vi "功能试验判定.vi"(7 "Result":refnum<vi>, 10 "判定参数":T1, 11 "XY曲线":cluster{"X":dbl[], "Y":dbl[]}[](array[cluster])) -> (2 "判定项长度":i32, 3 "OK？":bool)   [LabVIEW 2020]
uses:
  <userlib>/_MGI/1D Array/MGI Average/MGI Average (DBL[]).vi
panel:
  out "逆向平均值":dbl
  out "正向平均值":dbl
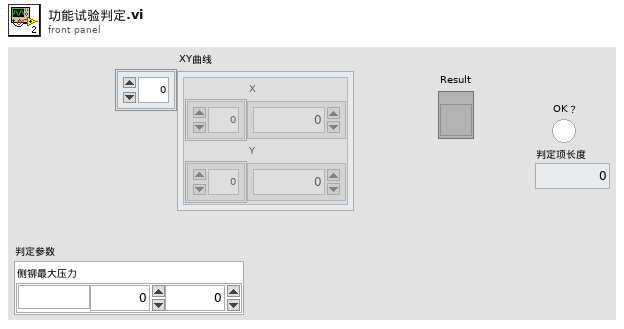
[diagram p1: front panel]
types:
  T1 = cluster{"侧铆最大压力":cluster{"单位":string, "下限":dbl, "上限":dbl}}
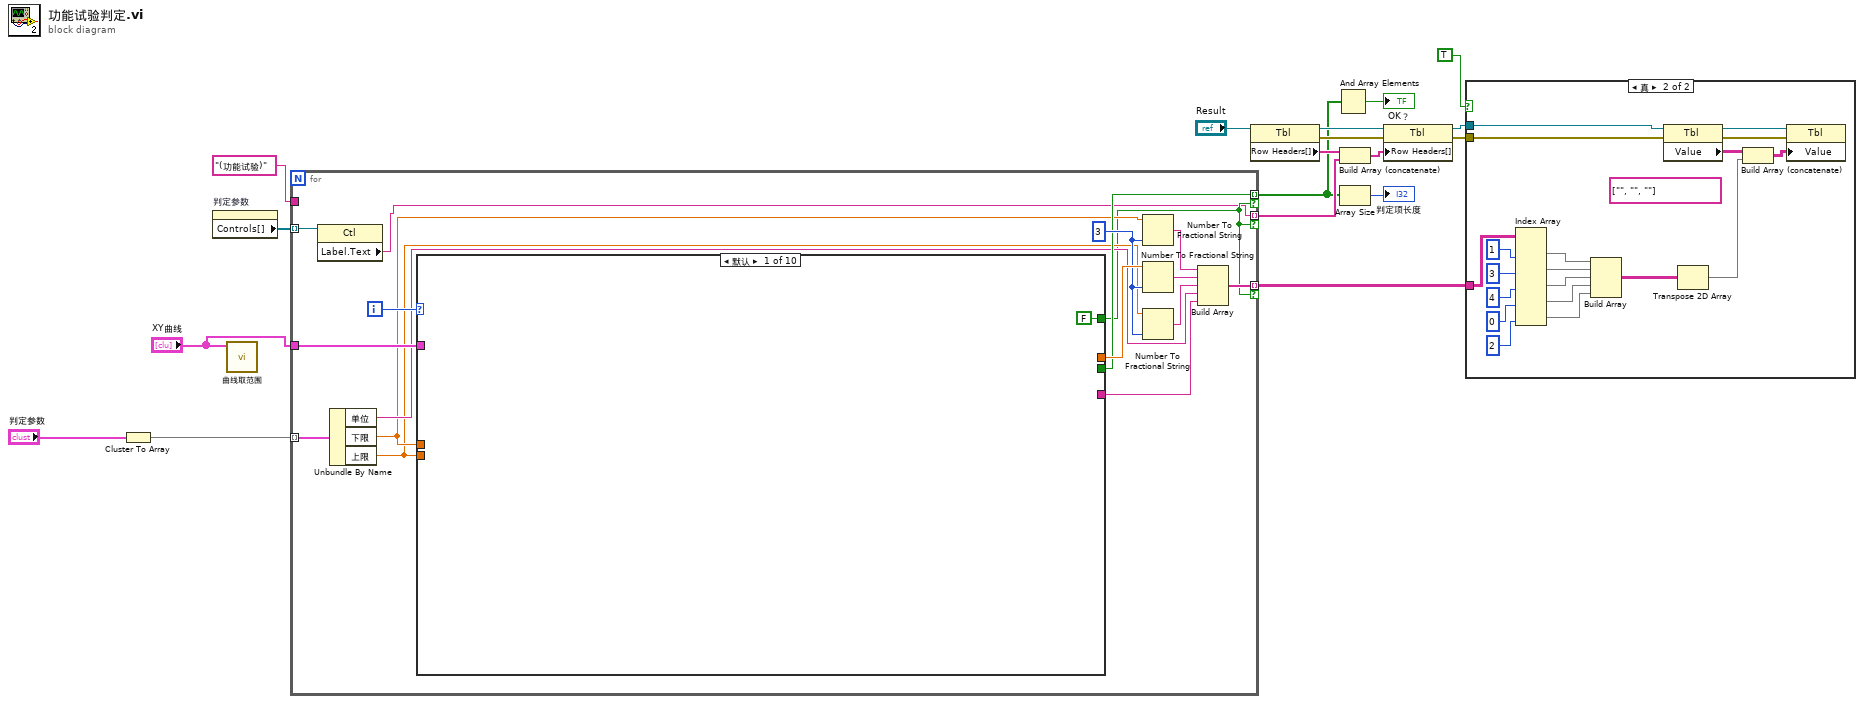
[diagram p0: block diagram]
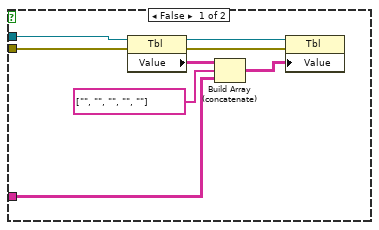
[diagram p2: hidden frame]
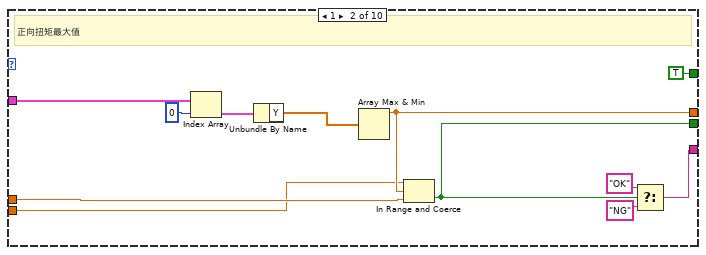
[diagram p3: hidden frame]
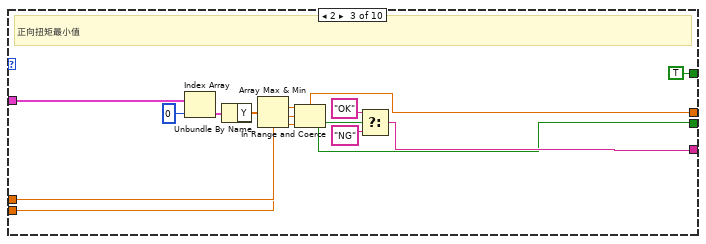
[diagram p4: hidden frame]
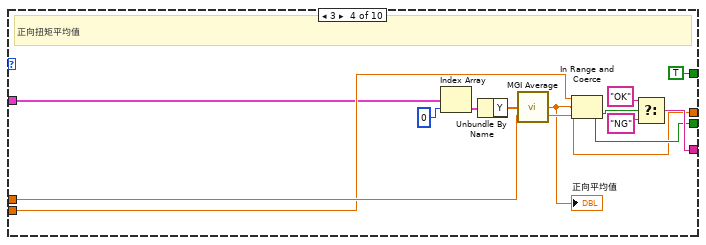
[diagram p5: hidden frame]
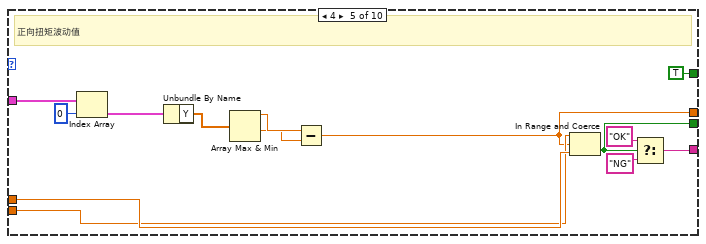
[diagram p6: hidden frame]
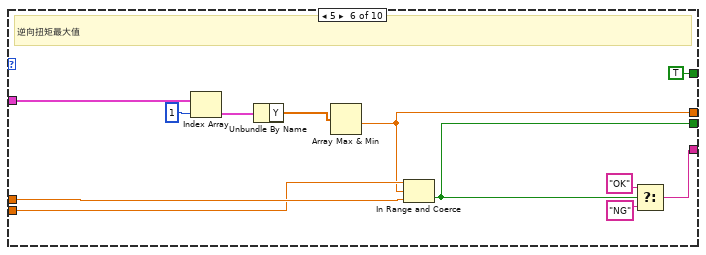
[diagram p7: hidden frame]
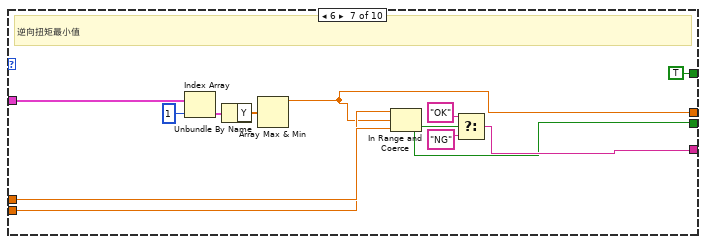
[diagram p8: hidden frame]
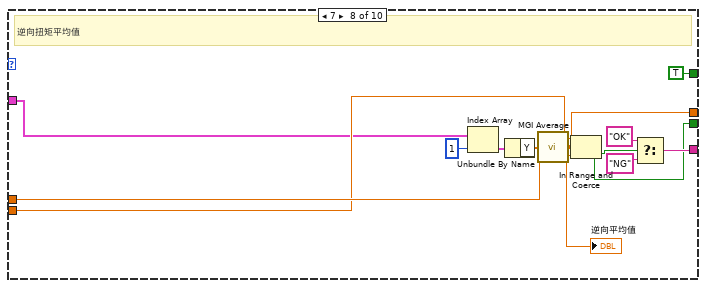
[diagram p9: hidden frame]
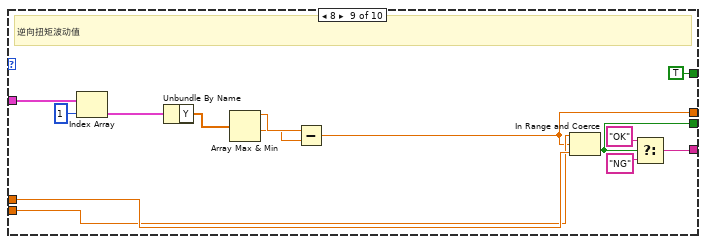
[diagram p10: hidden frame]
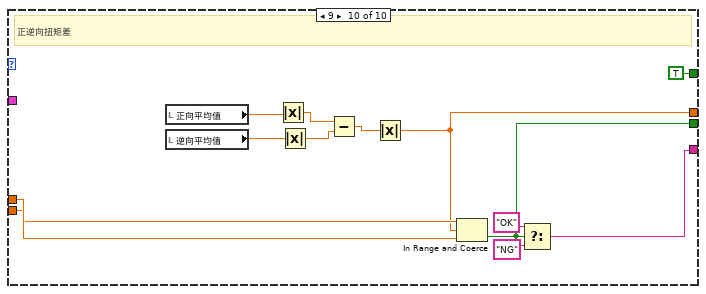
[diagram p11: hidden frame]
diagram:
  n1 = Cluster To Array(cluster="判定参数") -> (array=w18:cluster{"单位":string, "下限":dbl, "上限":dbl}[])
  n2 = property on="判定参数" class="Clust (严格)"() -> ("Controls[]"=w7:refnum<vi>[])  [unwired: 2 in, 2 out]
  n3 = call "曲线取范围.vi"("曲线In"="XY曲线") -> ()  [unwired: 10 in, 1 out]
  n4 = for {
    tunnel: w18 -> [w35] mode=indexing
    tunnel: w7 -> [w33] mode=indexing
    tunnel: "XY曲线" -> [w31]
    tunnel: [w25] -> w5 mode=indexing if=w20
    tunnel: [w21] -> w8 mode=indexing if=w20
    tunnel: [w19] -> w11 mode=indexing if=w20
    tunnel: "(功能试验)" ("Label.Text") -> [_]
    i -> [w34]
    w30 = i16 3 ("精度(6)")
    n5 = property class="Ctl"(reference=w33) -> ("Label.Text"=w19:string)  [unwired: 1 in, 2 out]
    n6 = Unbundle By Name(w35) -> ("单位"=w24:string, "下限"=w23:dbl, "上限"=w22:dbl)
    n7 = case shown="默认" w34 {
      tunnel: [_ w45 w51 w61 w73 w87 w99 w111 w123 w137] -> w32
      tunnel: w31 -> [_ w48 w60 w65 w79 w98 w110 w115 w129 _]
      tunnel: [_ w42 w56 w70 w84 w93 w106 w120 w134 w139] -> w26
      tunnel: [_ w41 w55 w69 w83 w92 w105 w119 w133 w138] -> w25
      tunnel: w23 -> [_ w40 w54 w68 w82 w91 w104 w118 w132 w146]
      tunnel: w22 -> [_ w39 w53 w67 w81 w90 w103 w117 w131 w145]
      tunnel: [FALSE TRUE TRUE TRUE TRUE TRUE TRUE TRUE TRUE TRUE] -> w20
      frame Default {
      }
      frame 1 {
        # "正向扭矩最大值"
        n8 = Index Array(array=w48, index=0 ("索引")) -> (element=w46:cluster{"X":dbl[], "Y":dbl[]})
        n9 = Unbundle By Name(w46) -> ("Y"=w37:dbl[])
        n10 = Array Max & Min(array=w37) -> (max value=w45:dbl)  [unwired: 3 out]
        n11 = In Range and Coerce(upper limit=w39, x=w45, lower limit=w40) -> (In Range?=w41:bool)  [unwired: 1 out]
        n12 = Select(t="OK", s=w41, f="NG") -> (s? t:f=w42:string)
      }
      frame 2 {
        # "正向扭矩最小值"
        n13 = Index Array(array=w60, index=0 ("索引")) -> (element=w59:cluster{"X":dbl[], "Y":dbl[]})
        n14 = Unbundle By Name(w59) -> ("Y"=w50:dbl[])
        n15 = Array Max & Min(array=w50) -> (min value=w51:dbl)  [unwired: 3 out]
        n16 = In Range and Coerce(upper limit=w53, x=w51, lower limit=w54) -> (In Range?=w55:bool)  [unwired: 1 out]
        n17 = Select(t="OK", s=w55, f="NG") -> (s? t:f=w56:string)
      }
      frame 3 {
        # "正向扭矩平均值"
        n18 = Index Array(array=w65, index=0 ("索引")) -> (element=w64:cluster{"X":dbl[], "Y":dbl[]})
        n19 = Unbundle By Name(w64) -> ("Y"=w63:dbl[])
        n20 = call-poly <userlib>:"MGI Average.vi"("Double[]"=w63) -> ("Average"=w61:dbl)  [unwired: 1 in]
        "正向平均值" <- w61
        n21 = In Range and Coerce(upper limit=w67, x=w61, lower limit=w68) -> (In Range?=w69:bool)  [unwired: 1 out]
        n22 = Select(t="OK", s=w69, f="NG") -> (s? t:f=w70:string)
      }
      frame 4 {
        # "正向扭矩波动值"
        n23 = Index Array(array=w79, index=0 ("索引")) -> (element=w78:cluster{"X":dbl[], "Y":dbl[]})
        n24 = Unbundle By Name(w78) -> ("Y"=w76:dbl[])
        n25 = Array Max & Min(array=w76) -> (max value=w75:dbl, min value=w74:dbl)  [unwired: 2 out]
        n26 = Subtract(x=w75, y=w74) -> (x-y=w73:dbl)
        n27 = In Range and Coerce(upper limit=w81, x=w73, lower limit=w82) -> (In Range?=w83:bool)  [unwired: 1 out]
        n28 = Select(t="OK", s=w83, f="NG") -> (s? t:f=w84:string)
      }
      frame 5 {
        # "逆向扭矩最大值"
        n29 = Index Array(array=w98, index=1 ("索引")) -> (element=w96:cluster{"X":dbl[], "Y":dbl[]})
        n30 = Unbundle By Name(w96) -> ("Y"=w88:dbl[])
        n31 = Array Max & Min(array=w88) -> (min value=w87:dbl)  [unwired: 3 out]
        n32 = In Range and Coerce(upper limit=w90, x=w87, lower limit=w91) -> (In Range?=w92:bool)  [unwired: 1 out]
        n33 = Select(t="OK", s=w92, f="NG") -> (s? t:f=w93:string)
      }
      frame 6 {
        # "逆向扭矩最小值"
        n34 = Index Array(array=w110, index=1 ("索引")) -> (element=w109:cluster{"X":dbl[], "Y":dbl[]})
        n35 = Unbundle By Name(w109) -> ("Y"=w101:dbl[])
        n36 = Array Max & Min(array=w101) -> (max value=w99:dbl)  [unwired: 3 out]
        n37 = In Range and Coerce(upper limit=w103, x=w99, lower limit=w104) -> (In Range?=w105:bool)  [unwired: 1 out]
        n38 = Select(t="OK", s=w105, f="NG") -> (s? t:f=w106:string)
      }
      frame 7 {
        # "逆向扭矩平均值"
        n39 = Index Array(array=w115, index=1 ("索引")) -> (element=w114:cluster{"X":dbl[], "Y":dbl[]})
        n40 = Unbundle By Name(w114) -> ("Y"=w113:dbl[])
        n41 = call-poly <userlib>:"MGI Average.vi"("Double[]"=w113) -> ("Average"=w111:dbl)  [unwired: 1 in]
        "逆向平均值" <- w111
        n42 = In Range and Coerce(upper limit=w117, x=w111, lower limit=w118) -> (In Range?=w119:bool)  [unwired: 1 out]
        n43 = Select(t="OK", s=w119, f="NG") -> (s? t:f=w120:string)
      }
      frame 8 {
        # "逆向扭矩波动值"
        n44 = Index Array(array=w129, index=1 ("索引")) -> (element=w128:cluster{"X":dbl[], "Y":dbl[]})
        n45 = Unbundle By Name(w128) -> ("Y"=w126:dbl[])
        n46 = Array Max & Min(array=w126) -> (max value=w125:dbl, min value=w124:dbl)  [unwired: 2 out]
        n47 = Subtract(x=w125, y=w124) -> (x-y=w123:dbl)
        n48 = In Range and Coerce(upper limit=w131, x=w123, lower limit=w132) -> (In Range?=w133:bool)  [unwired: 1 out]
        n49 = Select(t="OK", s=w133, f="NG") -> (s? t:f=w134:string)
      }
      frame 9 {
        # "正逆向扭矩差"
        n50 = local read "正向平均值"() -> (w144:dbl)
        n51 = local read "逆向平均值"() -> (w143:dbl)
        n52 = Absolute Value(x=w144) -> (abs(x)=w142:dbl)
        n53 = Absolute Value(x=w143) -> (abs(x)=w141:dbl)
        n54 = Subtract(x=w142, y=w141) -> (x-y=w140:dbl)
        n55 = Absolute Value(x=w140) -> (abs(x)=w137:dbl)
        n56 = In Range and Coerce(upper limit=w145, x=w137, lower limit=w146) -> (In Range?=w138:bool)  [unwired: 1 out]
        n57 = Select(t="OK", s=w138, f="NG") -> (s? t:f=w139:string)
      }
    }
    n58 = Number To Fractional String(number=w23, precision (6)=w30) -> (F-format string=w29:string)  [unwired: 2 in]
    n59 = Number To Fractional String(number=w32, precision (6)=w30) -> (F-format string=w28:string)  [unwired: 2 in]
    n60 = Number To Fractional String(number=w22, precision (6)=w30) -> (F-format string=w27:string)  [unwired: 2 in]
    n61 = Build Array(w29, w28, w27, w24, w26) -> (w21:string[])
  }
  n62 = property class="Tbl"(reference="Result") -> (reference out=w13:refnum<vi>, error out=w16:errorcluster, "Row Headers[]"=w9:string[])  [unwired: 1 in]
  n63 = And Array Elements(Boolean array=w5) -> (logical AND=→"OK？":bool)
  n64 = Build Array (concatenate)(w9, w11) -> (w12:string[])
  n65 = Array Size(array=w5) -> (size(s)=→"判定项长度":i32)
  n66 = property class="Tbl"(reference=w13, error in=w16, "Row Headers[]"=w12) -> (reference out=w14:refnum<vi>, error out=w15:errorcluster)
  n67 = case shown="真" TRUE {
    tunnel: w15 -> [w155 w174]
    tunnel: w14 -> [w152 w171]
    tunnel: w8 -> [w151 w163]
    frame False {
      n68 = property class="Tbl"(reference=w152, error in=w155) -> (reference out=w153:refnum<vi>, error out=w154:errorcluster, "Value"=w156:string[][])
      n69 = Build Array (concatenate)(w156, string[] ["", "", "", "", ""], w151) -> (w157:string[][])
      n70 = property class="Tbl"(reference=w153, error in=w154, "Value"=w157) -> ()  [unwired: 2 out]
    }
    frame True {
      (unwired) string[] ["", "", ""]
      n71 = Index Array(array=w163, index (col) #1=1 ("禁用的索引 (列)"), index (col) #2=3 ("索引 (列)"), index (col) #3=4 ("索引 (列)"), index (col) #4=0 ("索引 (列)"), index (col) #5=2 ("索引 (列)")) -> (element #1=w167:string[], element #2=w168:string[], element #3=w169:string[], element #4=w159:string[], element #5=w158:string[])  [unwired: 5 in]
      n72 = Build Array(w167, w168, w169, w159, w158) -> (w170:string[][])
      n73 = property class="Tbl"(reference=w171, error in=w174) -> (reference out=w172:refnum<vi>, error out=w173:errorcluster, "Value"=w175:string[][])
      n74 = Transpose 2D Array(2D array=w170) -> (transposed array=w162:string[][])
      n75 = Build Array (concatenate)(w175, w162) -> (w176:string[][])
      n76 = property class="Tbl"(reference=w172, error in=w173, "Value"=w176) -> ()  [unwired: 2 out]
    }
  }
